vi "GVSDataView SplitterShadow Moving Process.vi"(8 "DataView Index":i32, 9 "Bar_shadow ref":refnum<vi>, 10 "Mouse Pos":T1, 11 "SpliterMoveInfo":T2) -> ()   [LabVIEW 2013]
uses:
  GVSNew View Global.vi
  <vilib>/Utility/cursorutil.llb/Set Cursor (Icon Pict).vi
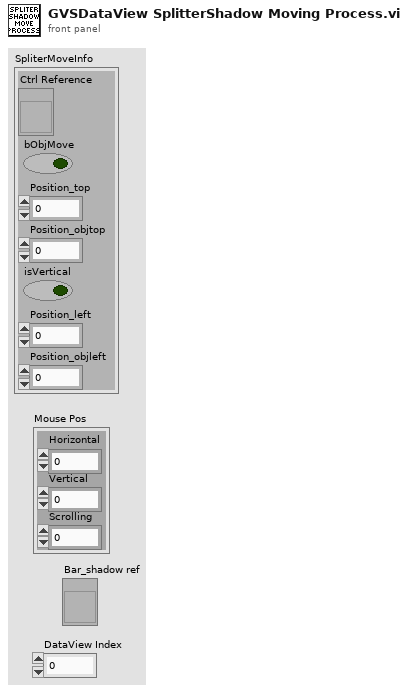
[diagram p1: front panel]
types:
  T1 = cluster{"Horizontal":i32, "Vertical":i32, "Scrolling":i32}
  T2 = cluster{"Ctrl Reference":refnum<vi>, "bObjMove":bool, "Position_top":i32, "Position_objtop":i32, "isVertical":bool, "Position_left":i32, "Position_objleft":i32}
  T3 = typedef "Graph Main Info Cluster.ctl" = cluster{"Selected_BarIdx":i32, "Selected_PanelIdx":i32, "Graph Main VIRef":refnum<vi>, "ToolBarClick":bool, "Spliter Ref Array":refnum<vi>[], "Panel Ref Array":refnum<vi>[], "Spliter_matrix":i32[][], "Panel_matrix":i32[][], "child_spliterIdx_matrix":i32[][], "split_pos_matrix":i32[][], "Title State":bool, "sQueueName":string, "Frame nID":i32, "Graph VIRef Array":cluster{"Graph VIRef":refnum<vi>, "Panel Idx":i32, "Frame VIRef":refnum<vi>, "Icon Ring":i32, "Graph Type":string}[], "View Type":string}
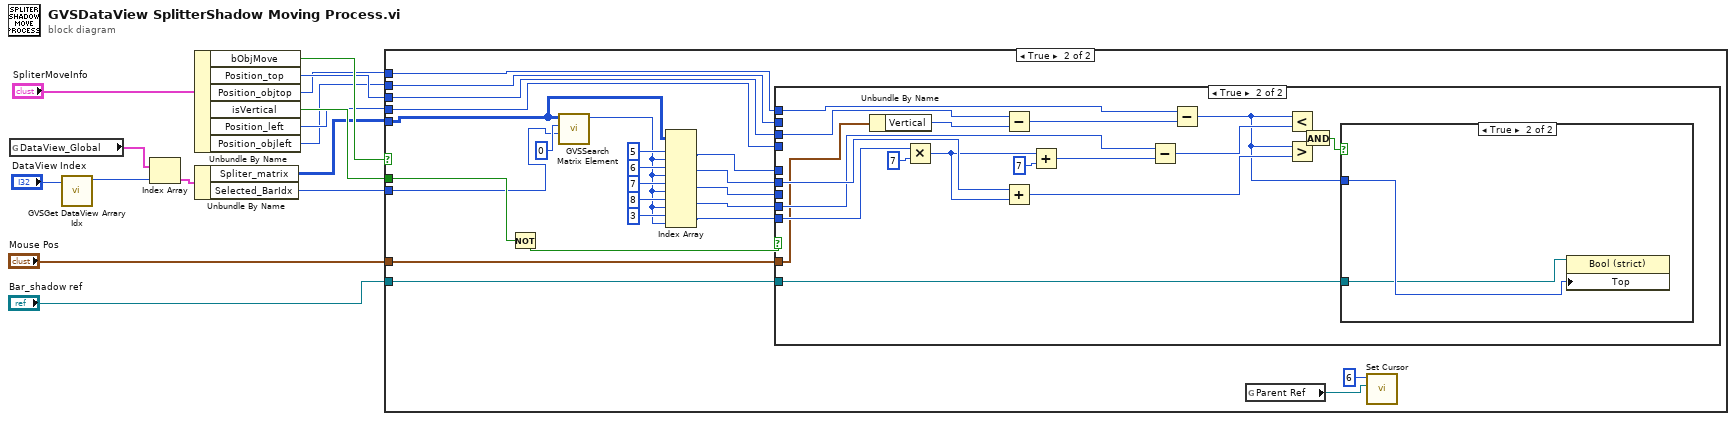
[diagram p0: block diagram]
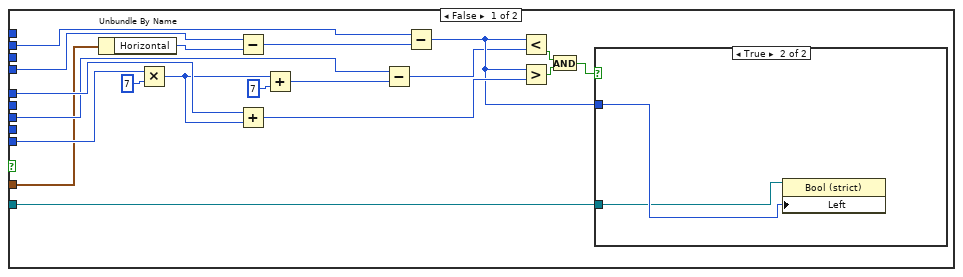
[diagram p3: hidden frame]
diagram:
  n1 = global read "GVSNew View Global.vi" "DataView_Global"() -> (w9:T3[])
  n2 = call "GVSGet DataView Arrary Idx.vi"("DataView Idx In"="DataView Index") -> ("DataView Arrary Idx out"=w1:i32)  [unwired: 10 in]
  n3 = Index Array(array=w9, index=w1) -> (element=w8:T3)
  n4 = Unbundle By Name("SpliterMoveInfo") -> ("bObjMove"=w15:bool, "Position_top"=w14:i32, "Position_objtop"=w13:i32, "isVertical"=w12:bool, "Position_left"=w11:i32, "Position_objleft"=w10:i32)
  n5 = Unbundle By Name(w8) -> ("Spliter_matrix"=w3:i32[][], "Selected_BarIdx"=w7:i32)
  n6 = case shown="True" w15 {
    tunnel: w14 -> [_ w39]
    tunnel: w13 -> [_ w38]
    tunnel: w12 -> [_ w35]
    tunnel: w11 -> [_ w37]
    tunnel: w10 -> [_ w36]
    tunnel: w3 -> [_ w24]
    tunnel: w7 -> [_ w33]
    tunnel: "Mouse Pos" -> [_ w31]
    tunnel: "Bar_shadow ref" -> [_ w30]
    frame False {
    }
    frame True {
      n7 = Not(x=w35) -> (.not. x?=w32:bool)
      n8 = call "GVSSearch Matrix Element.vi"("element"=w33, "index (row)"=0, "matrix in"=w24) -> ("index of element"=w23:i32)  [unwired: 8 in]
      n9 = Index Array(array=w24, index (row) #1=5 ("index (row)"), index (col) #1=w23, index (row) #2=6 ("index (row)"), index (col) #2=w23, index (row) #3=7 ("index (row)"), index (col) #3=w23, index (row) #4=8 ("index (row)"), index (col) #4=w23, index (row) #5=3 ("index (row)"), index (col) #5=w23) -> (element #1=w22:i32, element #2=w21:i32, element #3=w20:i32, element #4=w19:i32, element #5=w18:i32)
      n10 = case shown="True" w32 {
        tunnel: w39 -> [_ w79]
        tunnel: w38 -> [_ w78]
        tunnel: w37 -> [w56 _]
        tunnel: w36 -> [w55 _]
        tunnel: w22 -> [w54 _]
        tunnel: w20 -> [w50 _]
        tunnel: w21 -> [_ w75]
        tunnel: w19 -> [_ w73]
        tunnel: w18 -> [w46 w67]
        tunnel: w31 -> [w41 w62]
        tunnel: w30 -> [w40 w61]
        frame False {
          n11 = Unbundle By Name(w41) -> ("Horizontal"=w57:i32)
          n12 = Multiply(x=w46, y=7) -> (x*y=w43:i32)
          n13 = Subtract(x=w56, y=w57) -> (x-y=w58:i32)
          n14 = Add(x=w54, y=w43) -> (x+y=w53:i32)
          n15 = Add(x=w43, y=7) -> (x+y=w42:i32)
          n16 = Subtract(x=w50, y=w42) -> (x-y=w51:i32)
          n17 = Subtract(x=w55, y=w58) -> (x-y=w52:i32)
          n18 = Less?(x=w52, y=w51) -> (x < y?=w49:bool)
          n19 = Greater?(x=w52, y=w53) -> (0:w48:bool)
          n20 = And(x=w49, y=w48) -> (x .and. y?=w47:bool)
          n21 = case shown="True" w47 {
            tunnel: w52 -> [_ w60]
            tunnel: w40 -> [_ w59]
            frame False {
            }
            frame True {
              n22 = property class="Bool (strict)"(reference=w59, "Left"=w60) -> ()  [unwired: 1 in, 2 out]
            }
          }
        }
        frame True {
          n23 = Unbundle By Name(w62) -> ("Vertical"=w76:i32)
          n24 = Multiply(x=w67, y=7) -> (x*y=w65:i32)
          n25 = Subtract(x=w79, y=w76) -> (x-y=w77:i32)
          n26 = Add(x=w75, y=w65) -> (x+y=w74:i32)
          n27 = Add(x=w65, y=7) -> (x+y=w63:i32)
          n28 = Subtract(x=w73, y=w63) -> (x-y=w72:i32)
          n29 = Subtract(x=w78, y=w77) -> (x-y=w71:i32)
          n30 = Less?(x=w71, y=w72) -> (x < y?=w70:bool)
          n31 = Greater?(x=w71, y=w74) -> (0:w69:bool)
          n32 = And(x=w70, y=w69) -> (x .and. y?=w68:bool)
          n33 = case shown="True" w68 {
            tunnel: w71 -> [_ w81]
            tunnel: w61 -> [_ w80]
            frame False {
            }
            frame True {
              n34 = property class="Bool (strict)"(reference=w80, "Top"=w81) -> ()  [unwired: 1 in, 2 out]
            }
          }
        }
      }
      n35 = global read "GVSNew View Global.vi" "Parent Ref"() -> (w16:refnum<vi>)
      n36 = call-poly <vilib>:"Set Cursor.vi"("VI reference (current VI)"=w16, "icon"=u16 6) -> ()  [unwired: 1 in, 9 out]
    }
  }
